vi "Set Strain.vi"(6 "Channel":i32, 8 "error in (no error)":errorcluster, 9 "Slew (V/s)":dbl, 10 "Strain (V)":dbl, 11 "Instrument.Strain in":refnum<class "Instrument.Strain.lvclass">) -> (0 "error out":errorcluster, 3 "Instrument.Strain out":refnum<class "Instrument.Strain.lvclass">)   [LabVIEW 2019, in "Instrument.Strain.lvclass"]
uses:
  Instrument.Strain.lvclass
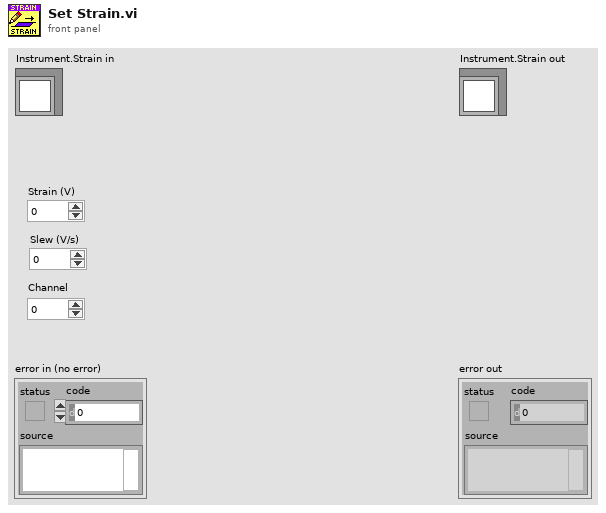
[diagram p1: front panel]
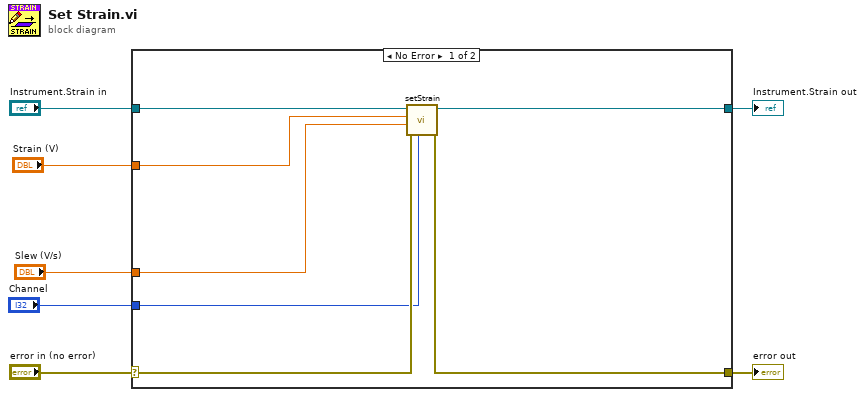
[diagram p0: block diagram]
diagram:
  n1 = case shown="No Error" "error in (no error)" {
    selector: "error in (no error)" -> [w10 w16]
    tunnel: [w8 w16] -> w6
    tunnel: [w13 w15] -> w4
    tunnel: "Instrument.Strain in" -> [w14 w15]
    tunnel: "Strain (V)" -> [w12 _]
    tunnel: "Slew (V/s)" -> [w11 _]
    tunnel: "Channel" -> [w9 _]
    frame No Error {
      n2 = call-dynamic "setStrain.vi"("Channel"=w9, "error in (no error)"=w10, "Slew (V/s)"=w11, "Strain (V)"=w12, "Instrument.Strain in"=w14) -> ("error out"=w8:errorcluster, "Instrument.Strain out"=w13:refnum<class "Instrument.Strain.lvclass">)  [unwired: 5 in]
    }
    frame Error {
    }
  }
  "error out" <- w6
  "Instrument.Strain out" <- w4
